vi "sCMOSStand_Analog.vi"(4 "stand Z vol Backward samp":cluster{"Fs":dbl, "#s":dbl}={"Fs"=500000.0, "#s"=68421.0}, 6 "stand Z vol Acquisition samp":cluster{"Fs":dbl, "#s":dbl}={"Fs"=500000.0, "#s"=131579.0}, 8 "error in (no error)":errorcluster, 10 "stand Z vol Acquisition time (s)":dbl=0.2631578947368421, 11 "Steps per volume":dbl=25.0) -> (0 "error out":errorcluster, 2 "sCMOSStand":waveform(dbl))   [LabVIEW 2018]
uses:
  <vilib>/Waveform/WDTOps.llb/WDT Append Waveforms DBL.vi
  <vilib>/measure/NI_MABase.lvlib
panel:
  out "Preview":waveform(dbl)(graph)
  out "sCMOS blank waveform":waveform(dbl)(graph)={"t0"=timestamp(0 s since 1904-01-01), "dt"=1e-06, "Y"=array[400000 elements]}
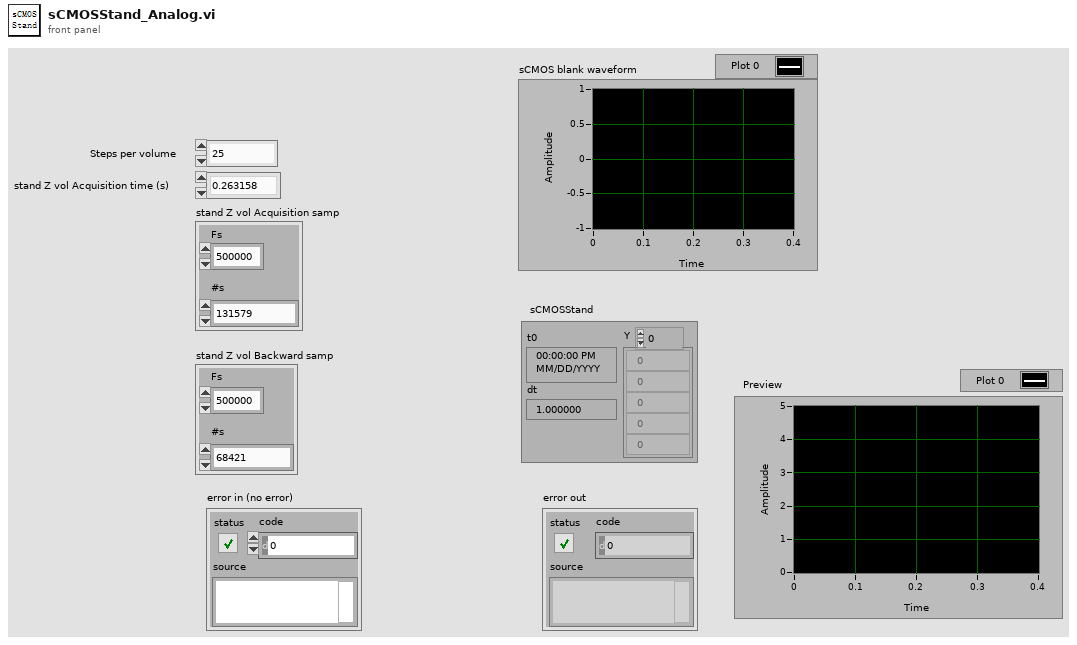
[diagram p1: front panel]
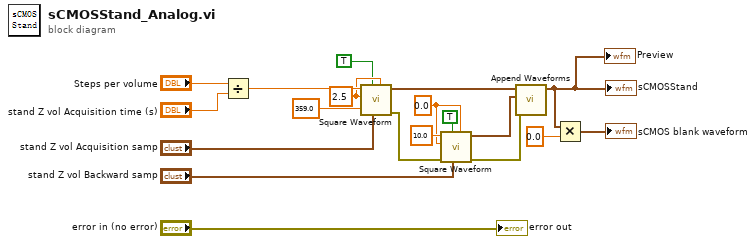
[diagram p0: block diagram]
diagram:
  w13 = 0.0 ("offset")
  w17 = 2.5 ("amplitude")
  n1 = Divide(x="Steps per volume", y="stand Z vol Acquisition time (s)") -> (x/y=w18:dbl)
  n2 = call <vilib>:"Square Waveform.vi"("offset"=w17, "sampling info"="stand Z vol Acquisition samp", "reset signal"=TRUE, "phase"=359.0, "amplitude"=w17, "frequency"=w18) -> ("error out"=w11:errorcluster, "signal out"=w9:waveform(dbl))  [unwired: 4 in]
  n3 = call <vilib>:"Square Waveform.vi"("offset"=w13, "sampling info"="stand Z vol Backward samp", "reset signal"=TRUE, "error in (no error)"=w11, "amplitude"=w13, "frequency"=10.0) -> ("error out"=w8:errorcluster, "signal out"=w10:waveform(dbl))  [unwired: 4 in]
  n4 = call-poly <vilib>:"Append Waveforms.vi"("error in (no error)"=w8, "waveform B"=w10, "waveform A"=w9) -> ("waveform out"=w1:waveform(dbl))  [unwired: 7 in, 1 out]
  "sCMOSStand" <- w1
  "Preview" <- w1
  n5 = Multiply(x=w1, y=0.0) -> (x*y=→"sCMOS blank waveform":waveform(dbl))
  "error out" <- "error in (no error)"
